vi "listbox_alternate_colors.vi"(6 "Recolor? (T)":bool=TRUE, 8 "error_in":errorcluster, 10 "item_names":string[][](array[string]), 11 "listbox_ref":refnum<vi>) -> (0 "error_out":errorcluster)   [LabVIEW 2020]
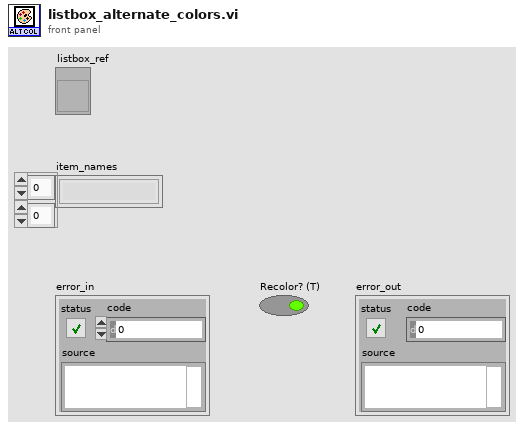
[diagram p1: front panel]
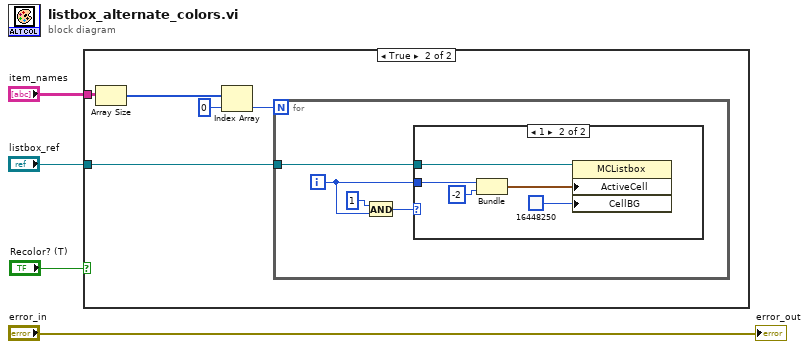
[diagram p0: block diagram]
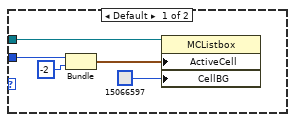
[diagram p3: hidden frame]
diagram:
  n1 = case shown="True" "Recolor? (T)" {
    tunnel: "item_names" -> [_ w6]
    tunnel: "listbox_ref" -> [_ w5]
    frame False {
    }
    frame True {
      n2 = Array Size(array=w6) -> (size(s)=w7:i32[])
      n3 = Index Array(array=w7, index=0) -> (element=w8:i32)
      n4 = for {
        N: w8 -> [_]
        tunnel: w5 -> [w13]
        i -> [w10]
        n5 = And(x=1, y=w10) -> (x .and. y?=w11:i32)
        n6 = case shown="1" w11 {
          tunnel: w13 -> [w18 w22]
          tunnel: w10 -> [w14 w23]
          frame Default {
            n7 = Bundle(w14, -2) -> (w16:cluster{i32, i32})  [unwired: 1 in]
            n8 = property on="Property Node" class="MCListbox"(reference=w18, "ActiveCell"=w16, "CellBG"=u32 15066597) -> ()  [unwired: 1 in, 2 out]
          }
          frame 1 {
            n9 = Bundle(w23, -2) -> (w20:cluster{i32, i32})  [unwired: 1 in]
            n10 = property on="Property Node" class="MCListbox"(reference=w22, "ActiveCell"=w20, "CellBG"=u32 16448250) -> ()  [unwired: 1 in, 2 out]
          }
        }
      }
    }
  }
  "error_out" <- "error_in"
